vi "Display.vi"() -> ()   [LabVIEW 2010]
panel:
  in  "stop":bool
  in  "Axis":u16(ring) items=["X"]
  out "Status":string
  in  "Tab Control":T1(tab)
  out "Position Command":dbl
  out "Position Feedback":dbl
  out "Prog Pos Command":dbl
  out "Prog Pos Feedback":dbl
  out "Velocity Command":dbl
  out "Velocity Feedback":dbl
  out "Current Command":sgl
  out "Current Feedback":sgl
  out "Amplifier Temp":sgl
  out "Pos Fbk Auxiliary":dbl
  out "Analog Input 0":dbl
  out "Analog Input 1":dbl
  out "Analog Output 0":dbl
  out "Analog Output 1":dbl
  out "Digital Input 0":bool[](array[boolean])
  out "Digital Input 1":bool[](array[boolean])
  out "Digital Input 2":bool[](array[boolean])
  out "Digital Output 0":bool[](array[boolean])
  out "Digital Output 1":bool[](array[boolean])
  out "Digital Output 2":bool[](array[boolean])
  out "Axis Fault (bits)":T2
  out "Axis Status (bits)":T3
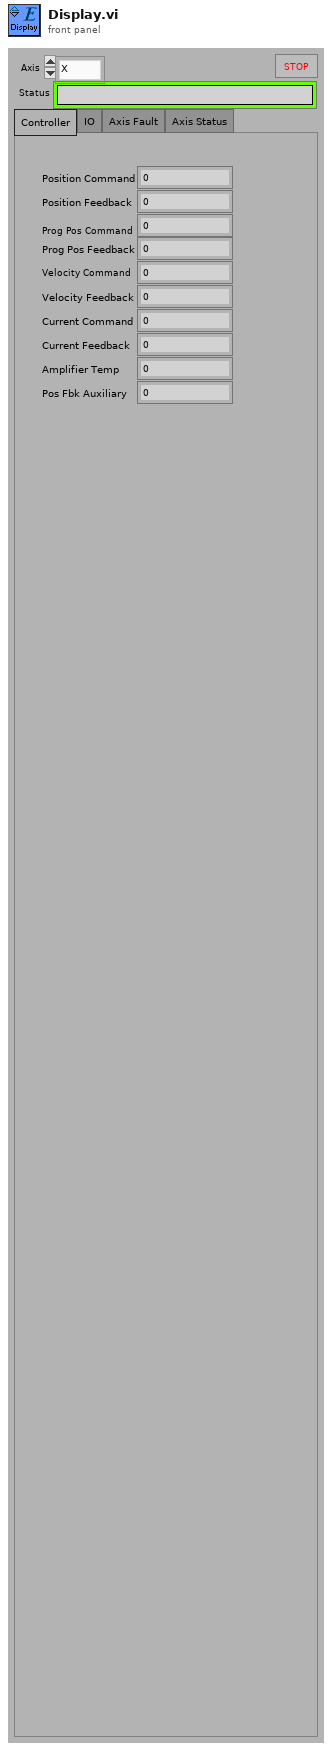
[diagram p1: front panel]
types:
  T1 = enum32{"Controller", "IO", "Axis Fault", "Axis Status"}
  T2 = cluster{"AmplifierFault":bool, "AmplifierTemperatureFault":bool, "CcwEndOfTravelLimitFault":bool, "CcwSoftwareLimitFault":bool, "CommunicationLostFault":bool, "CwEndOfTravelLimitFault":bool, "CwSoftwareLimitFault":bool, "EmergencyStopFault":bool, "EncoderFault":bool, "ExternalFault":bool, "FeedbackScalingFault":bool, "HallSensorFault":bool, "MarkerSearchFault":bool, "MaxVelocityCommandFault":bool, "MotorTemperatureFault":bool, "None":bool, "OverCurrentFault":bool, "PositionErrorFault":bool, "PositionFeedbackFault":bool, "PowerSupplyFault":bool, "VelocityErrorFault":bool, "VelocityFeedbackFault":bool, "VoltageClampFault":bool}
  T3 = cluster{"AccelerationPhase":bool, "AutofocusActive":bool, "BrakeOutput":bool, "CalibrationActive":bool, "CalibrationEnabled":bool, "CcwEndOfTravelLimitInput":bool, "CommandShapingFilterDone":bool, "CosineEncoderError":bool, "CurrentClamp":bool, "CwEndOfTravelLimitInput":bool, "DecelerationPhase":bool, "EmergencyStopInput":bool, "Enabled":bool, "GantryMasterActive":bool, "GantryModeActive":bool, "HallAInput":bool, "HallBInput":bool, "HallCInput":bool, "Homed":bool, "HomeLimitInput":bool, "Homing":bool, "InPosition":bool, "InPosition2":bool, "JoystickControl":bool, "MarkerInput":bool, "MasterMotionSuppressed":bool, "MasterSlaveControl":bool, "MotionIsCw":bool, "MoveActive":bool, "None":bool, "PositionCaptureActive":bool, "ServoControl":bool, "SineEncoderError":bool}
  T4 = cluster{"new reference":refnum<k24>, "Event Callback":refnum<k27>, "ControllerDiagPacket":refnum<user-event>, "Event Registration Refnum":refnum<event-registration>}
  T5 = typedef "AxisDiagPacket.ctl" = cluster{"Axis Name":string, "Acceleration Command":dbl, "Amplifier Temperature":sgl, "Analog Input 0":dbl, "Analog Input 1":dbl, "Analog Output 0":dbl, "Analog Output 1":dbl, "Axis Fault (num)":i32, "Axis Fault (str)":string, "Axis Fault (bits)":cluster{"AmplifierFault":bool, "AmplifierTemperatureFault":bool, "CcwEndOfTravelLimitFault":bool, "CcwSoftwareLimitFault":bool, "CommunicationLostFault":bool, "CwEndOfTravelLimitFault":bool, "CwSoftwareLimitFault":bool, "EmergencyStopFault":bool, "EncoderFault":bool, "ExternalFault":bool, "FeedbackScalingFault":bool, "HallSensorFault":bool, "MarkerSearchFault":bool, "MaxVelocityCommandFault":bool, "MotorTemperatureFault":bool, "None":bool, "OverCurrentFault":bool, "PositionErrorFault":bool, "PositionFeedbackFault":bool, "VelocityErrorFault":bool, "VelocityFeedbackFault":bool, "VoltageClampFault":bool, "PowerSupplyFault":bool}, "Axis Status (num)":i32, "Axis Status (str)":string, "Axis Status (bits)":cluster{"AccelerationPhase":bool, "AutofocusActive":bool, "BrakeOutput":bool, "CalibrationActive":bool, "CalibrationEnabled":bool, "CcwEndOfTravelLimitInput":bool, "CommandShapingFilterDone":bool, "CosineEncoderError":bool, "CurrentClamp":bool, "CwEndOfTravelLimitInput":bool, "DecelerationPhase":bool, "EmergencyStopInput":bool, "Enabled":bool, "GantryMasterActive":bool, "GantryModeActive":bool, "HallAInput":bool, "HallBInput":bool, "HallCInput":bool, "Homed":bool, "HomeLimitInput":bool, "Homing":bool, "InPosition":bool, "InPosition2":bool, "JoystickControl":bool, "MarkerInput":bool, "MasterMotionSuppressed":bool, "MasterSlaveControl":bool, "MotionIsCw":bool, "MoveActive":bool, "None":bool, "PositionCaptureActive":bool, "ServoControl":bool, "SineEncoderError":bool}, "Current Command":sgl, "Current Error":sgl, "Current Feedback":sgl, "Digital Input 0":i32, "Digital Input 1":i32, "Digital Input 2":i32, "Digital Output 0":i32, "Digital Output 1":i32, "Digital Output 2":i32, "Position Feedback Auxiliary":dbl, "Position Command":dbl, "Position Error":dbl, "Position Feedback":dbl, "Program Position Command":dbl, "Program Position Error":dbl, "Program Position Feedback":dbl, "Velocity Command":dbl, "Velocity Error":dbl, "Velocity Feedback":dbl}
  T6 = cluster{"AmplifierFault":bool, "AmplifierTemperatureFault":bool, "CcwEndOfTravelLimitFault":bool, "CcwSoftwareLimitFault":bool, "CommunicationLostFault":bool, "CwEndOfTravelLimitFault":bool, "CwSoftwareLimitFault":bool, "EmergencyStopFault":bool, "EncoderFault":bool, "ExternalFault":bool, "FeedbackScalingFault":bool, "HallSensorFault":bool, "MarkerSearchFault":bool, "MaxVelocityCommandFault":bool, "MotorTemperatureFault":bool, "None":bool, "OverCurrentFault":bool, "PositionErrorFault":bool, "PositionFeedbackFault":bool, "VelocityErrorFault":bool, "VelocityFeedbackFault":bool, "VoltageClampFault":bool, "PowerSupplyFault":bool}
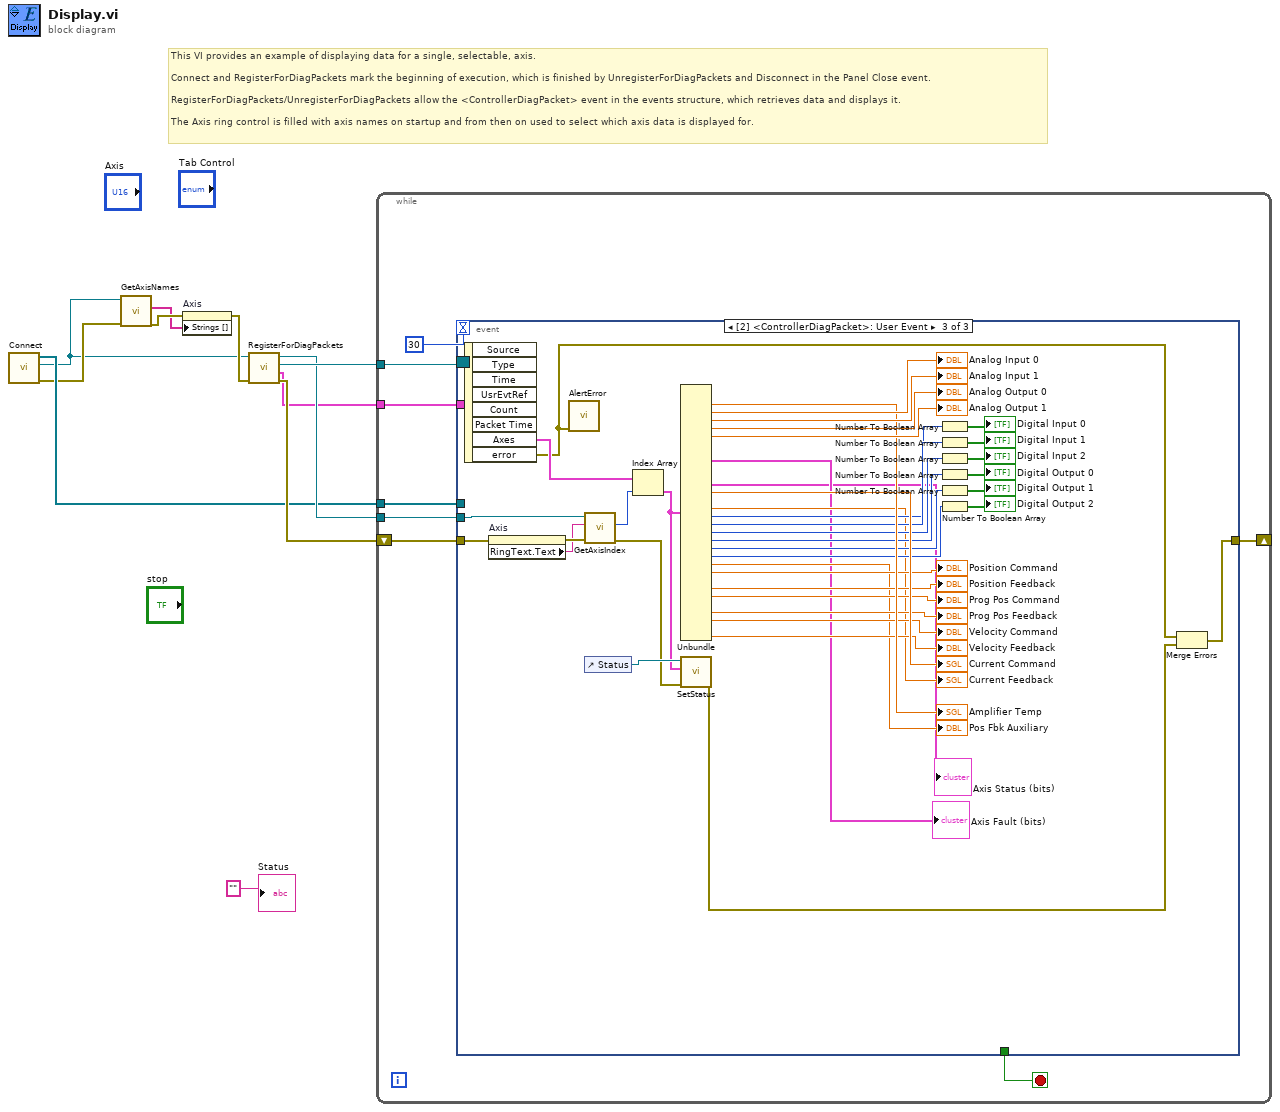
[diagram p0: block diagram]
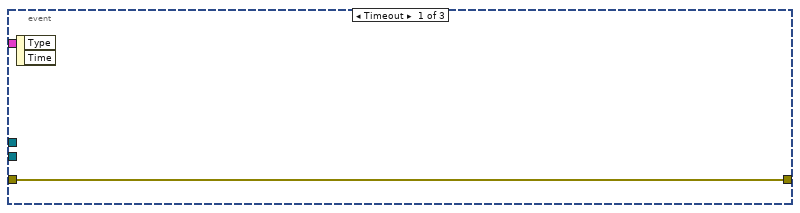
[diagram p2: hidden frame]
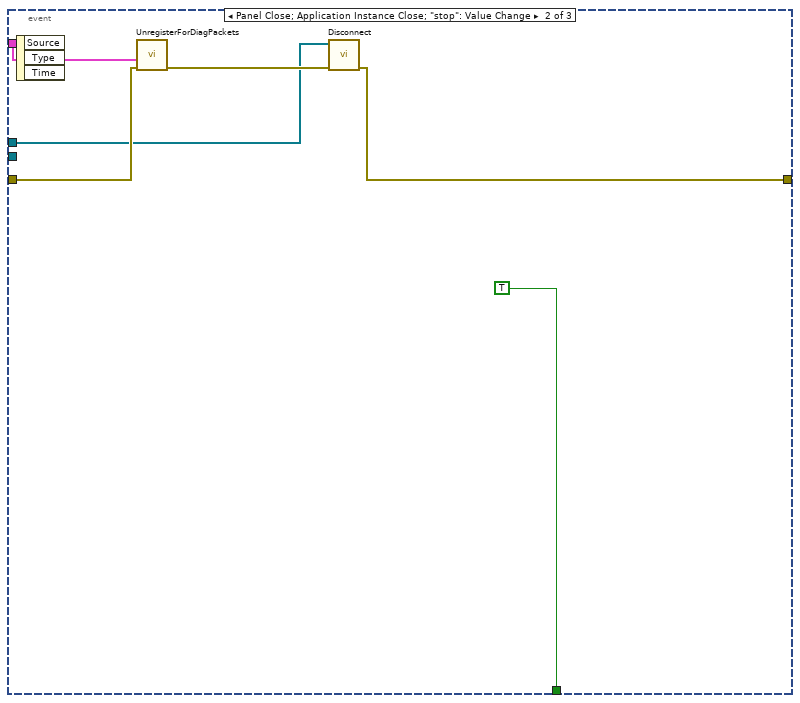
[diagram p3: hidden frame]
diagram:
  # "This VI provides an example of displaying data for a single, selectable, axis. \n\nConnect and RegisterForDiagPackets mark the beginning of execution, which is finished by UnregisterForDiagPackets and Disconnect in the Panel Close event.\n\nRegisterForDiagPackets/UnregisterForDiagPackets allow the <ControllerDiagPacket> event in the events structure, which retrieves data and displays it.\n\nThe Axis ring control is filled with axis names on startup and from then on used to select which axis data is displayed for."
  n1 = call "Connect.vi"() -> ("error out"=w4:errorcluster, "controller"=w3:refnum<k24>, "controllers"=w7:refnum<k24>[])  [unwired: 9 in]
  n2 = call "GetAxisNames.vi"("error in (no error)"=w4, "controller in"=w3) -> ("error out"=w5:errorcluster, "axis names"=w2:string[])  [unwired: 7 in, 1 out]
  n3 = property on="Axis" class="Ring (strict)"(error in=w5, "Strings []"=w2) -> (error out=w6:errorcluster)  [unwired: 1 in, 1 out]
  n4 = call "RegisterForDiagPackets.vi"("error in (no error)"=w6, "Controller in"=w3) -> ("error out"=w9:errorcluster, "Even Metadata"=w1:T4, "Event Registration Refnum"=w11:refnum<event-registration>, "Controller out"=w10:refnum<k24>)  [unwired: 5 in]
  n5 = while {
    tunnel: w11 -> [w19]
    tunnel: w10 -> [w18]
    shift-right: [w14] -> _
    shift-left: w9 -> [w17]
    tunnel: w7 -> [w13]
    tunnel: w1 -> [w12]
    stop <- w16 stop-if-true
    n6 = event shown="[2] <ControllerDiagPacket>: User Event" {
      selector: w19 -> [_ _ _]
      dyn-events: _ -> [_ _ _]
      timeout: 30 -> [_ _ _]
      tunnel: w18 -> [_ _ w54]
      tunnel: w17 -> [w20 w26 w53]
      tunnel: [_ TRUE _] -> w16
      tunnel: [w20 w23 w62] -> w14
      tunnel: w13 -> [_ w22 _]
      tunnel: w12 -> [_ w21 _]
      event Timeout {
        n7 = event-data() -> ()  [unwired: 1 in, 2 out]
      }
      event Panel Close; Application Instance Close; "stop": Value Change {
        n8 = event-data() -> ()  [unwired: 1 in, 3 out]
        n9 = call "UnregisterForDiagPackets.vi"("error in (no error)"=w26, "Even Metadata"=w21) -> ("error out"=w25:errorcluster)  [unwired: 9 in]
        n10 = call "Disconnect.vi"("error in (no error)"=w25, "controllers"=w22) -> ("error out"=w23:errorcluster)  [unwired: 9 in]
      }
      event User Event {
        n11 = event-data() -> ("Axes"=w66:T5[], "error"=w61:errorcluster)  [unwired: 1 in, 6 out]
        n12 = property on="Axis" class="Ring (strict)"(error in=w53) -> (error out=w52:errorcluster, "RingText.Text"=w51:string)  [unwired: 1 in, 1 out]
        n13 = call "AlertError.vi"("error in (no error)"=w61) -> ()  [unwired: 10 in, 1 out]
        n14 = call "GetAxisIndex.vi"("error in (no error)"=w52, "axis name"=w51, "controller in"=w54) -> ("error out"=w49:errorcluster, "axis index"=w50:i32)  [unwired: 6 in, 1 out]
        n15 = control-ref of="Status"() -> (w65:refnum<vi>)
        n16 = Index Array(array=w66, index=w50) -> (element=w64:T5)
        n17 = Unbundle(w64) -> ("Amplifier Temperature"=→"Amplifier Temp":sgl, "Analog Input 0"=→"Analog Input 0":dbl, "Analog Input 1"=→"Analog Input 1":dbl, "Analog Output 0"=→"Analog Output 0":dbl, "Analog Output 1"=→"Analog Output 1":dbl, "Axis Fault (bits)"=→"Axis Fault (bits)":T6, "Axis Status (bits)"=→"Axis Status (bits)":T3, "Current Command"=→"Current Command":sgl, "Current Feedback"=→"Current Feedback":sgl, "Digital Input 0"=w30:i32, "Digital Input 1"=w31:i32, "Digital Input 2"=w32:i32, "Digital Output 0"=w33:i32, "Digital Output 1"=w34:i32, "Digital Output 2"=w35:i32, "Position Feedback Auxiliary"=→"Pos Fbk Auxiliary":dbl, "Position Command"=→"Position Command":dbl, "Position Feedback"=→"Position Feedback":dbl, "Program Position Command"=→"Prog Pos Command":dbl, "Program Position Feedback"=→"Prog Pos Feedback":dbl, "Velocity Command"=→"Velocity Command":dbl, "Velocity Feedback"=→"Velocity Feedback":dbl)  [unwired: 10 out]
        n18 = call "SetStatus.vi"("error in (no error)"=w49, "AxisDiagPacket"=w64, "Status string"=w65) -> ("error out"=w63:errorcluster)  [unwired: 8 in]
        n19 = Number To Boolean Array(number=w30) -> (Boolean array=→"Digital Input 0":bool[])
        n20 = Number To Boolean Array(number=w31) -> (Boolean array=→"Digital Input 1":bool[])
        n21 = Number To Boolean Array(number=w32) -> (Boolean array=→"Digital Input 2":bool[])
        n22 = Number To Boolean Array(number=w33) -> (Boolean array=→"Digital Output 0":bool[])
        n23 = Number To Boolean Array(number=w34) -> (Boolean array=→"Digital Output 1":bool[])
        n24 = Number To Boolean Array(number=w35) -> (Boolean array=→"Digital Output 2":bool[])
        n25 = Merge Errors(w61, w63) -> (w62:errorcluster)
      }
    }
  }
  "Status" <- "" ("Status")
